vi "Increment N_Groups.vi"(8 "error in":errorcluster, 11 "TDMS in":refnum<class "TDMS.lvclass">) -> (0 "error out":errorcluster, 2 "new group number":u16, 3 "TDMS out":refnum<class "TDMS.lvclass">)   [LabVIEW 2011, in "TDMS.lvclass"]
uses:
  TDMS.lvclass
  TDMS.lvclass/TDMS.ctl
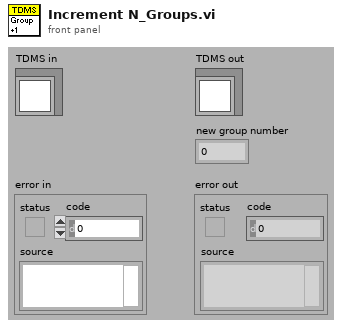
[diagram p1: front panel]
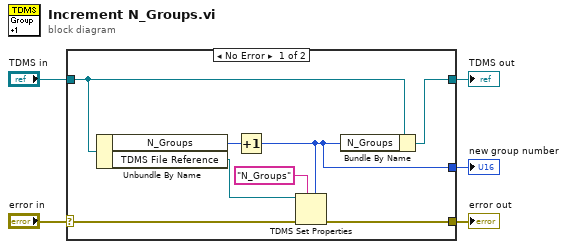
[diagram p0: block diagram]
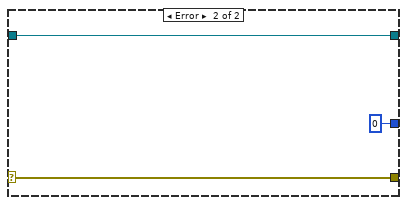
[diagram p2: hidden frame]
diagram:
  n1 = case shown="No Error" "error in" {
    selector: "error in" -> [w7 w15]
    tunnel: [w6 w15] -> w4
    tunnel: [w13 w16] -> w2
    tunnel: "TDMS in" -> [w12 w16]
    tunnel: [w8 u16 0] -> w1
    frame No Error {
      n2 = Unbundle By Name(w12) -> ("N_Groups"=w11:u16, "TDMS File Reference"=w10:refnum<k34>)
      n3 = Increment(x=w11) -> (x+1=w8:u16)
      n4 = TDMS Set Properties(5:w8, 7:"N_Groups", 8:w7, 11:w10) -> (0:w6:errorcluster)  [unwired: 2 in, 3 out]
      n5 = Bundle By Name(cluster=w12, "N_Groups"=w8) -> (w13:refnum<class "TDMS.lvclass">)
    }
    frame Error {
    }
  }
  "error out" <- w4
  "TDMS out" <- w2
  "new group number" <- w1
